vi "tsdb_load_flexray_db.vi"(8 "error in (no error)":errorcluster caption="错误输入（无错误）", 9 "Channels":i32[](array[numeric]), 10 "AFRFile":path=path "C:/Users/DYR/Desktop/M110.dbc", 11 "路径输入":path) -> (0 "error out":errorcluster caption="错误输出", 1 "AId out":i32, 2 "function return":i32, 3 "路径输出":path)   [LabVIEW 2014]
doc: "Function Introduction: Loading Flexray Database\nCall location\nInput parameter 1:\n AFliepath Fliepath\nParameter 2:\n ASupportedChannels SupportedChannels\nParameter 3:\n AId Id\nReturn value==0: Setting successful\nOther: Failed, check the error type based on the error code"
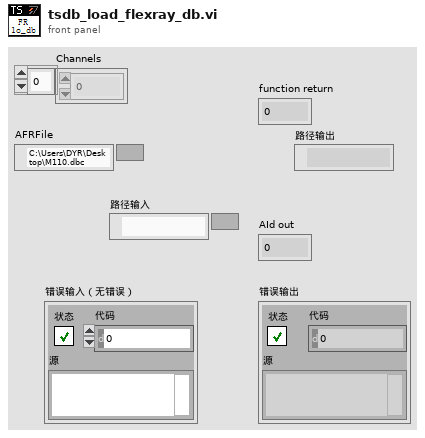
[diagram p1: front panel]
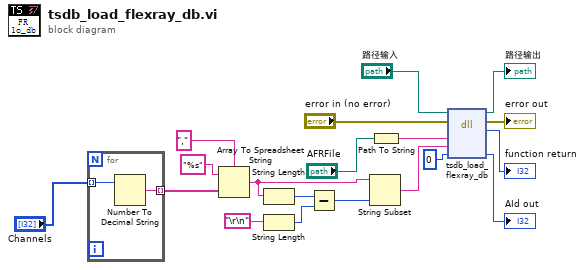
[diagram p0: block diagram]
diagram:
  n1 = for {
    tunnel: "Channels" -> [w21] mode=indexing
    tunnel: [w20] -> w6 mode=indexing
    n2 = Number To Decimal String(number=w21) -> (decimal integer string=w20:string)  [unwired: 1 in]
  }
  n3 = Array To Spreadsheet String(delimiter (Tab)="," ("delimiter"), array=w6, 3:"%s" ("format string")) -> (spreadsheet string=w8:string)
  n4 = String Length(string=w8) -> (length=w10:i32)
  n5 = String Length(string="\r\n") -> (length=w9:i32)
  n6 = Subtract(x=w10, y=w9) -> (x-y=w7:i32)
  n7 = String Subset(string=w8, length (rest)=w7) -> (substring=w4:string)  [unwired: 1 in]
  n8 = Path To String(path="AFRFile") -> (string=w2:string)
  n9 = dll-call lib="D:/Work/LabVIEW Code/TSMaster Labview SDK/LabVIEW/LabVIEW-TSMasterAPI_CLN/TSMasterAPI_LabVIEW-2024-10-08 14-20-13/Not_organized_vi/TSMaster.*" fn="tsdb_load_flexray_db"(path in="路径输入", error in="error in (no error)", "AFRFile"=w2, "ASupportedChannels"=w4, "AId"=0) -> (path out=→"路径输出":path, error out=→"error out":errorcluster, "返回类型"=→"function return":i32, "AId"=→"AId out":i32)  [unwired: 3 in]
